vi "SDR_AttPara.vi"(10 "TX1衰减":u16=50 caption="dB" max=90 step=1, 11 "ChannelSelection":enum16{"TxCh1", "TxCh2"}(ring)) -> (3 "AttPara":string)   [LabVIEW 2015]
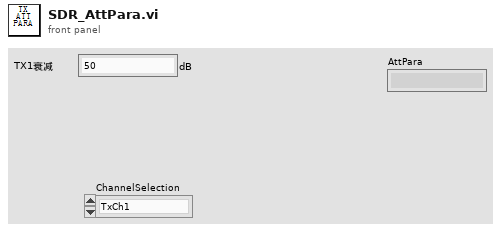
[diagram p1: front panel]
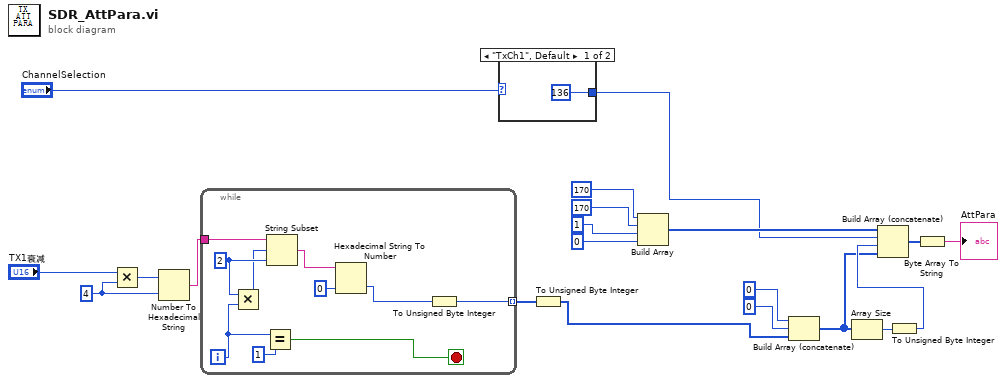
[diagram p0: block diagram]
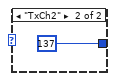
[diagram p2: hidden frame]
diagram:
  w18 = i16 4 ("宽度(-)")
  n1 = Multiply(x="TX1衰减", y=w18) -> (x*y=w17:u16)
  n2 = Number To Hexadecimal String(1:w18, 2:w17) -> (0:w20:string)
  n3 = while {
    tunnel: w20 -> [w28]
    tunnel: [w21] -> w19 mode=indexing
    i -> [w27]
    stop <- w29 stop-if-true
    w26 = 2 ("长度（剩余）")
    n4 = Multiply(x=w26, y=w27) -> (x*y=w25:i32)
    n5 = Equal?(x=w27, y=1) -> (x = y?=w29:bool)
    n6 = String Subset(string=w28, offset (0)=w25, length (rest)=w26) -> (substring=w24:string)
    n7 = Hexadecimal String To Number(string=w24, default (0uL)=u8 0 ("默认(0 U32)")) -> (number=w22:u8)  [unwired: 2 out]
    n8 = To Unsigned Byte Integer(number=w22) -> (unsigned 8bit integer=w21:u8)
  }
  n9 = case shown="\"TxCh1\", Default" "ChannelSelection" {
    tunnel: [u8 136 u8 137] -> w9
    frame "TxCh1", Default {
    }
    frame "TxCh2" {
    }
  }
  n10 = To Unsigned Byte Integer(number=w19) -> (unsigned 8bit integer=w10:u8[])
  n11 = Build Array(u8 170, u8 170, u8 1, u8 0) -> (w11:u8[])
  n12 = Build Array (concatenate)(u8 0, u8 0, w10) -> (w4:u8[])
  n13 = Array Size(array=w4) -> (size(s)=w6:i32)
  n14 = To Unsigned Byte Integer(number=w6) -> (unsigned 8bit integer=w5:u8)
  n15 = Build Array (concatenate)(w11, w9, w5, w4) -> (w3:u8[])
  n16 = Byte Array To String(unsigned byte array=w3) -> (string=→"AttPara":string)
